vi "Create New File.vi"(1 "Event Name":string, 2 "OK Button":bool) -> (0 "concatenated string":string)   [LabVIEW 2014]
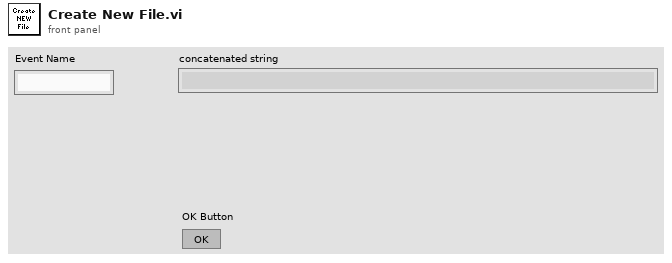
[diagram p1: front panel]
types:
  T1 = enum16{"open", "replace", "create", "open or create", "replace or create", "replace or create with confirmation"}
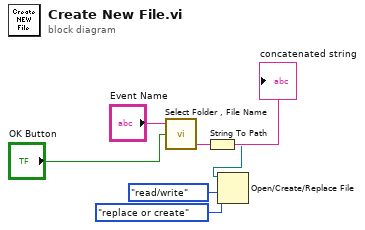
[diagram p0: block diagram]
diagram:
  n1 = call "Select Folder , File Name.vi"("OK Button"="OK Button", "File Name"="Event Name") -> ("concatenated string"=w5:string)
  "concatenated string" <- w5
  n2 = String To Path(string=w5) -> (path=w4:path)
  n3 = Open/Create/Replace File(file path (use dialog)=w4, operation (0:open)=T1."replace or create", access (0:read/write)=enum16{"read/write", "read-only", "write-only"}."read/write") -> ()  [unwired: 3 in, 3 out]
